vi "Construct_multipart_response_variant.vi"(0 "command":T3=enum."configure_rf", 1 "Status":T2, 5 "parameters (JSON)":string="{\"invalid\":1}", 7 "datatype":T1, 9 "data in":variant, 11 "error in (no error)":errorcluster) -> (3 "command_str":string="invalid_command", 4 "Multipart message":string[](array[string]), 14 "Debug info":string, 15 "error out":errorcluster)   [LabVIEW 2019, in "mmW_commands.lvlib"]
uses:
  TypeDefs/commands.ctl
  TypeDefs/response status.ctl
  commands/typedefs/datatypes_.ctl
  mmW_commands.lvlib
panel:
  out "type (none)":string="none"
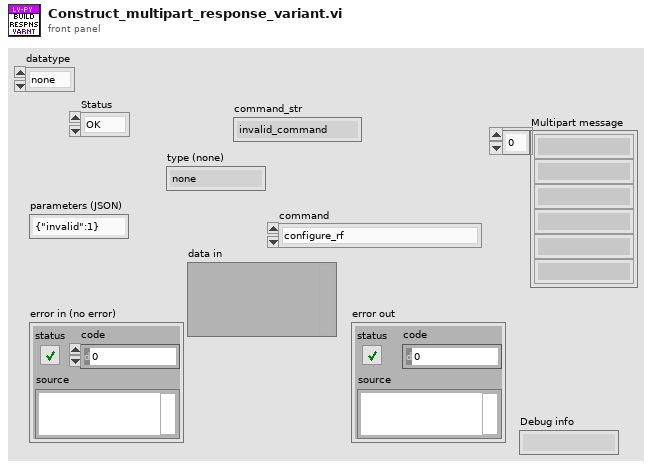
[diagram p1: front panel]
types:
  T1 = typedef "mmW_commands.lvlib/datatypes_.ctl" = enum16{"none", "string", "interleaved_I16", "interleaved_I32", "I16_array", "I32_array", "JSONstring"}
  T2 = typedef "mmW_commands.lvlib/response status.ctl" = enum16{"OK", "Error", "Warning", "Unknown"}
  T3 = typedef "mmW_commands.lvlib/commands.ctl" = enum16{"configure_fs", "configure_rf", "configure_trigger", "equalization_enable", "equalization_start", "lo_sync_enable", "equalization_stop", "get_instrument_status", "get_versions", "initialize_hw", "pop_rx", "set_log_level", "Shutdown", "start", "start_instrument_app", "stop", "trans", "transceive", "trigger_burst", "trigger_sync_enable", "Write TX", "resp_generic", "resp_waveform", "send_trigger", "fetch", "transceive2"}
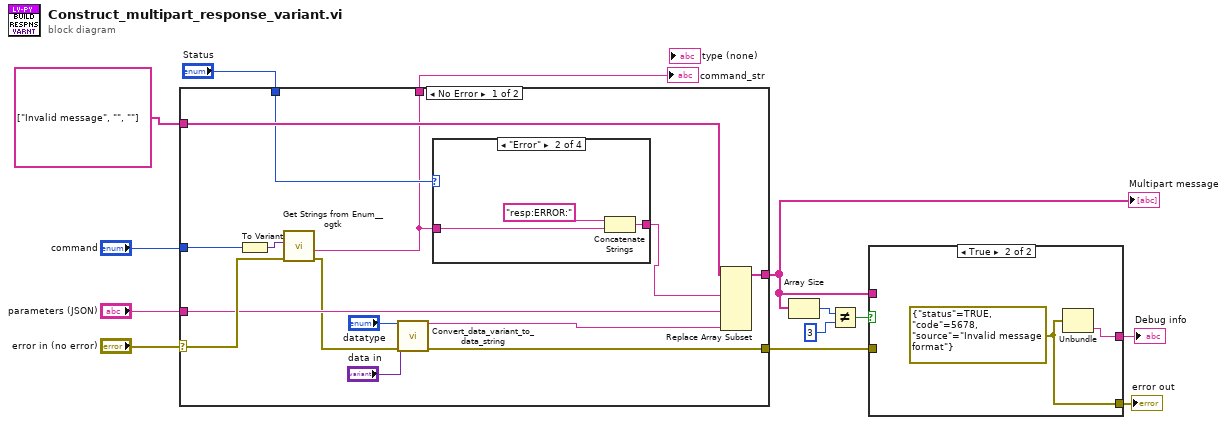
[diagram p0: block diagram]
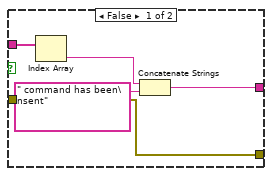
[diagram p2: hidden frame]
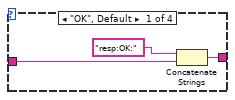
[diagram p3: hidden frame]
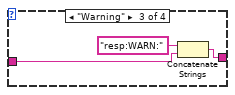
[diagram p4: hidden frame]
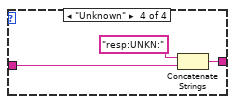
[diagram p5: hidden frame]
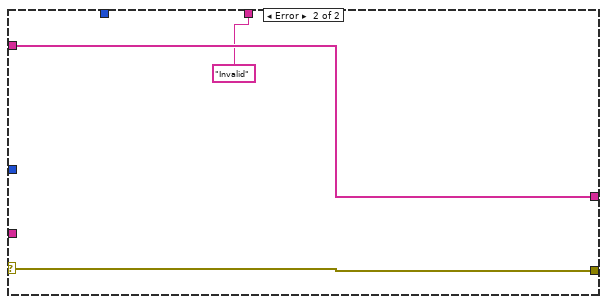
[diagram p6: hidden frame]
diagram:
  n1 = case shown="No Error" "error in (no error)" {
    selector: "error in (no error)" -> [w23 w41]
    tunnel: "parameters (JSON)" -> [w19 _]
    tunnel: [w17 w41] -> w6
    tunnel: [w27 w42] -> w5
    tunnel: string[] ["Invalid message", "", ""] -> [w26 w42]
    tunnel: "command" -> [w24 _]
    tunnel: [w21 "Invalid" ("String Value")] -> w2
    tunnel: "Status" -> [w22 _]
    frame No Error {
      n2 = To Variant(anything=w24) -> (Variant=w25:variant)
      n3 = call <userlib>:"Get Strings from Enum__ogtk.vi"("error in (no error)"=w23, "Enum"=w25) -> ("error out"=w18:errorcluster, "String Value"=w21:string)  [unwired: 6 in, 2 out]
      n4 = call "Convert_data_variant_to_data_string.vi"("datatype"="datatype", "data in"="data in", "error in (no error)"=w18) -> ("String"=w16:string, "error out"=w17:errorcluster)  [unwired: 11 in]
      n5 = case shown="\"Error\"" w22 {
        tunnel: w21 -> [w30 w33 w35 w38]
        tunnel: [w29 w31 w36 w39] -> w20
        frame "OK", Default {
          n6 = Concatenate Strings("resp:OK:" ("string"), w30) -> (w29:string)
        }
        frame "Error" {
          n7 = Concatenate Strings("resp:ERROR:" ("string"), w33) -> (w31:string)
        }
        frame "Warning" {
          n8 = Concatenate Strings("resp:WARN:" ("string"), w35) -> (w36:string)
        }
        frame "Unknown" {
          n9 = Concatenate Strings("resp:UNKN:" ("string"), w38) -> (w39:string)
        }
      }
      n10 = Replace Array Subset(array=w26, new element #1=w20, new element #2=w19, new element #3=w16) -> (w27:string[])  [unwired: 3 in]
    }
    frame Error {
    }
  }
  "Multipart message" <- w5
  "command_str" <- w2
  n11 = Array Size(array=w5) -> (size(s)=w10:i32)
  n12 = Not Equal?(x=w10, y=3) -> (x != y?=w8:bool)
  n13 = case shown="True" w8 {
    tunnel: [w47 w49] -> w7
    tunnel: w6 -> [w47 _]
    tunnel: w5 -> [w46 _]
    tunnel: [w43 w48] -> w4
    frame False {
      n14 = Index Array(array=w46) -> (element=w45:string)  [unwired: 1 in]
      n15 = Concatenate Strings(w45, " command has been\nsent" ("string")) -> (w43:string)
    }
    frame True {
      w49 = errorcluster {"status"=TRUE, "code"=5678, "source"="Invalid message format"} ("s? t:f")
      n16 = Unbundle(w49) -> ("source"=w48:string)  [unwired: 2 out]
    }
  }
  "error out" <- w7
  "Debug info" <- w4
